vi "enable.vi"(8 "error in (no error)":errorcluster, 11 "GenericEmissionSensor in":refnum<class "DetectorYK090623DAQmxAnalog.lvclass">) -> (0 "error out":errorcluster, 3 "GenericEmissionSensor out":refnum<class "DetectorYK090623DAQmxAnalog.lvclass">)   [LabVIEW 2010, in "DetectorYK090623DAQmxAnalog.lvclass"]
uses:
  DetectorYK090623DAQmxAnalog.lvclass
  DetectorYK090623DAQmxAnalog.lvclass/DetectorYK090623DAQmxAnalog.ctl
  AnalogOut/AnalogOutDL101207DAQmx/AnalogOutDL101207DAQmx/AnalogOutDL101207DAQmx.lvclass
  GenericDetector/GenericDetector/GenericDetector.lvclass
  common/classes/ErrorController/ErrorController/class_data.vi
  common/classes/ErrorController/ErrorController/ErrorController.lvclass
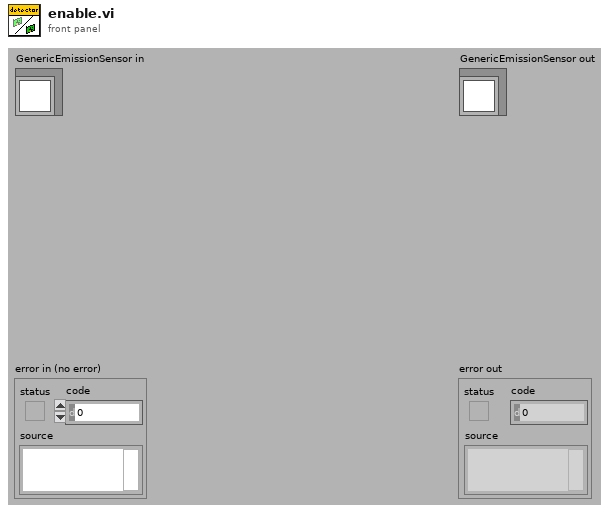
[diagram p1: front panel]
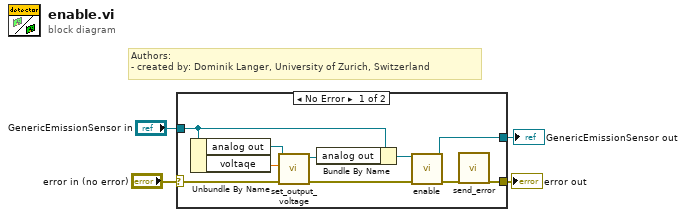
[diagram p0: block diagram]
diagram:
  # "Authors: \n- created by: Dominik Langer, University of Zurich, Switzerland"
  n1 = case shown="No Error" "error in (no error)" {
    selector: "error in (no error)" -> [w13 w16]
    tunnel: [w5 w16] -> w4
    tunnel: [w14 w15] -> w3
    tunnel: "GenericEmissionSensor in" -> [w8 w15]
    frame No Error {
      n2 = Unbundle By Name(w8) -> ("analog out"=w10:refnum<class "AnalogOutDL101207DAQmx.lvclass">, "voltaqe"=w11:dbl[unit])
      n3 = call-dynamic "set_output_voltage.vi"("error in (no error)"=w13, "output value"=w11, "DAQmxAnalogOut in"=w10) -> ("error out"=w12:errorcluster, "DAQmxAnalogOut out"=w9:refnum<class "AnalogOutDL101207DAQmx.lvclass">)  [unwired: 7 in]
      n4 = Bundle By Name(cluster=w8, "analog out"=w9) -> (w7:refnum<class "DetectorYK090623DAQmxAnalog.lvclass">)
      n5 = call-parent "enable.vi"("error in (no error)"=w12, "GenericEmissionSensor in"=w7) -> ("error out"=w6:errorcluster, "GenericEmissionSensor out"=w14:refnum<class "DetectorYK090623DAQmxAnalog.lvclass">)  [unwired: 8 out]
      n6 = call "send_error.vi"("error in (no error)"=w6) -> ("error out"=w5:errorcluster)  [unwired: 10 in]
    }
    frame Error {
    }
  }
  "error out" <- w4
  "GenericEmissionSensor out" <- w3
